vi "dfd_Get Filter Group Delay.vi"(5 "output option\n(T: FLP)":bool=TRUE, 6 "fs [Hz]":dbl=1.0 format="%.2f", 7 "freq points [Hz]":dbl[](array[numeric]) format="%.2f", 8 "error in (no error)":errorcluster, 11 "filter in":T1={"mSRate_Fs"=1.0, "mSRate_Version"="1.0", "mSRate_Comments"="", "mSRate_OrgCoef"={"type"=enum."Undefined", "gain"=1.0, "coef a (k)"=[], "coef b (v)"=[]}, "mSRate_CurCoef"={"type"=enum."Undefined", "gain"=1.0, "coef a (k)"=[], "coef b (v)"=[]}, "mSRate_Quantized?"=FALSE, "mSRate_QCoef"={"type"=enum."Undefined", "gain"=1.0, "coef a (k)"=[], "coef b (v)"=[]}, "mSRate_QSettings"=[], "mSRate_Order"=0, "mSRate_Scaling"={"mSRate_ScaleByPowerOf2?"=FALSE, "mSRate_ScaleType"=enum."No Norm"}} {"mSRate_QSettings"."source" items=["Coef a/k"=0, "Coef b/v"=7, "Input"=1, "Output"=2, "Multiplicand"=3, "Product"=4, "Sum"=5, "Delay"=6, "Gain"=8]}) -> (0 "error out":errorcluster, 3 "group delay":dbl[](array[numeric]) format="%.2f")   [LabVIEW 2017, in "NI_DigFilterLicensed.lvlib"]
uses:
  <vilib>/addons/Digital Filter Design/NI_DigFilterLicensed.lvlib
  <vilib>/addons/Digital Filter Design/_Objects.llb/DFD Filter Obj.ctl
  <vilib>/addons/Digital Filter Design/_Objects.llb/DFD Filter Coef.ctl
  <vilib>/addons/Digital Filter Design/_Objects.llb/DFD Filter Structure Type Selector.ctl
  <vilib>/addons/Digital Filter Design/_Objects.llb/dfd_Internal Quantization Settings.ctl
  <vilib>/addons/Digital Filter Design/_Objects.llb/dfd_Internal Quantization Srcs.ctl
  <vilib>/addons/Digital Filter Design/_Objects.llb/DFD Coef Norm Type.ctl
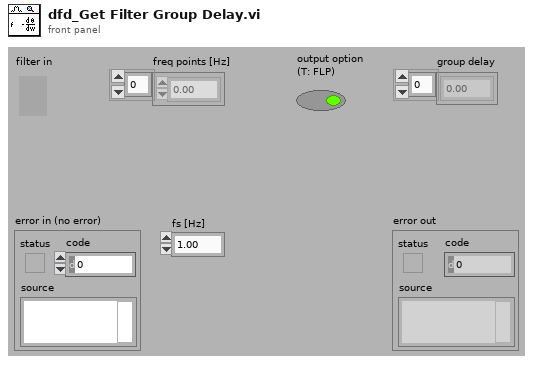
[diagram p1: front panel]
types:
  T1 = typedef "NI_DigFilterLicensed.lvlib/DFD Filter Obj.ctl" = cluster{"mSRate_Fs":dbl, "mSRate_Version":string, "mSRate_Comments":string, "mSRate_OrgCoef":T2, "mSRate_CurCoef":T2, "mSRate_Quantized?":bool, "mSRate_QCoef":T2, "mSRate_QSettings":T4[], "mSRate_Order":i32, "mSRate_Scaling":cluster{"mSRate_ScaleByPowerOf2?":bool, "mSRate_ScaleType":T6}}
  T2 = typedef "NI_DigFilterLicensed.lvlib/DFD Filter Coef.ctl" = cluster{"type":T3, "gain":dbl, "coef a (k)":dbl[], "coef b (v)":dbl[]}
  T3 = typedef "NI_DigFilterLicensed.lvlib/DFD Filter Structure Type Selector.ctl" = enum16{"Undefined", "FIR Direct Form", "FIR Direct Form Transposed", "FIR Symmetric", "FIR Antisymmetric", "IIR Direct Form I", "IIR Direct Form I Transposed", "IIR Direct Form II", "IIR Direct Form II Transposed", "IIR Cascaded Second Order Sections Form I", "IIR Cascaded Second Order Sections Form I Transposed", "IIR Cascaded Second Order Sections Form II", "IIR Cascaded Second Order Sections Form II Transposed", "Lattice Allpass (basic sections)", "Lattice Allpass (one multiplier sections)", "Lattice Allpass (normalized sections)", "Lattice AR (basic sections)", "Lattice AR (one multiplier sections)", "Lattice AR (normalized sections)", "Lattice MA (minimum phase)", "Lattice MA (maximum phase)", "Lattice ARMA (basic sections)", "Lattice ARMA (one multiplier sections)", "Lattice ARMA (normalized sections)"}
  T4 = typedef "NI_DigFilterLicensed.lvlib/dfd_Internal Quantization Settings.ctl" = cluster{"source":T5, "wl":i16, "iwl":i16, "overflow mode":enum16{"Saturation", "Wrap"}, "rounding mode":enum16{"Nearest", "Truncation"}, "signed?":bool}
  T5 = typedef "NI_DigFilterLicensed.lvlib/dfd_Internal Quantization Srcs.ctl" = u16
  T6 = typedef "NI_DigFilterLicensed.lvlib/DFD Coef Norm Type.ctl" = enum16{"No Norm", "Time Domain 1-Norm", "Time Domain 2-Norm", "Time Domain Inf-Norm"}
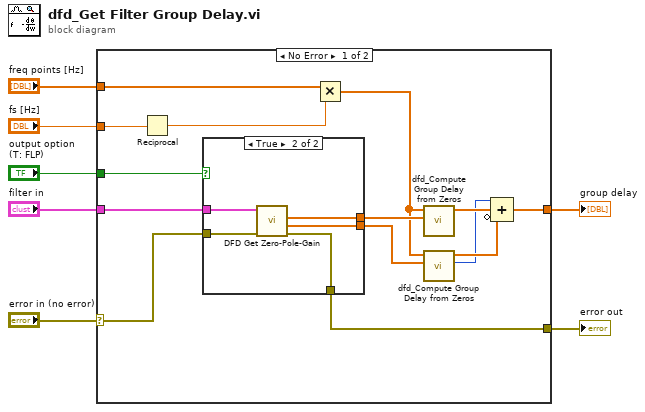
[diagram p0: block diagram]
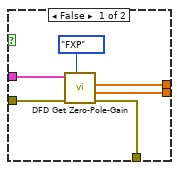
[diagram p2: hidden frame]
diagram:
  n1 = case shown="No Error" "error in (no error)" {
    selector: "error in (no error)" -> [w13 w33]
    tunnel: "freq points [Hz]" -> [w12 _]
    tunnel: "fs [Hz]" -> [w17 _]
    tunnel: "filter in" -> [w15 _]
    tunnel: "output option\n(T: FLP)" -> [w11 _]
    tunnel: [w9 _] -> w3
    tunnel: [w10 w33] -> w2
    frame No Error {
      n2 = Reciprocal(x=w17) -> (1/x=w14:dbl)
      n3 = case shown="True" w11 {
        tunnel: [w25 w32] -> w19
        tunnel: [w24 w31] -> w18
        tunnel: w15 -> [w27 w30]
        tunnel: w13 -> [w26 w29]
        tunnel: [w23 w28] -> w10
        frame False {
          n4 = call <vilib>:"DFD Get Zero-Pole-Gain.vi"("type (FLP)"=enum16{"FLP", "FXP"}."FXP", "error in (no error)"=w26, "filter in"=w27) -> ("error out"=w23:errorcluster, "poles"=w24:cdb[], "zeroes"=w25:cdb[])  [unwired: 6 out]
        }
        frame True {
          n5 = call <vilib>:"DFD Get Zero-Pole-Gain.vi"("error in (no error)"=w29, "filter in"=w30) -> ("error out"=w28:errorcluster, "poles"=w31:cdb[], "zeroes"=w32:cdb[])  [unwired: 7 out]
        }
      }
      n6 = Multiply(x=w12, y=w14) -> (x*y=w16:dbl[])
      n7 = call <vilib>:"dfd_Compute Group Delay from Zeros.vi"("roots"=w19, "freq points"=w16) -> ("group delay"=w21:dbl[])  [unwired: 1 in, 8 out]
      n8 = call <vilib>:"dfd_Compute Group Delay from Zeros.vi"("roots"=w18, "freq points"=w16) -> ("# zero root"=w8:i32, "group delay"=w20:dbl[])  [unwired: 2 in, 6 out]
      n9 = Compound Arithmetic op=ADD(w8, w21, invert w20) -> (w9:dbl[])
    }
    frame Error {
    }
  }
  "error out" <- w2
  "group delay" <- w3
